vi "DimostratoreCalibrazioni.vi"() -> ()   [LabVIEW 2019]
uses:
  TypeDef/SlugExpiration.ctl
  ByteGSAPIBase/ByteGSAPIBase.lvclass
  TypeDef/CalibrationStates.ctl
  ByteGSAPIBase/FetchCalibration/Converted_Slug_Cluster.ctl
  ByteGSAPIBase/Instruments/Instruments.ctl
  ByteGSAPIBase/CalibrationMeasurements/BodyCalibrazioneMisure.ctl
  aa47c742-c095-4670-bf1f-6b28e4309cef.vi
  <vilib>/numeric/Random Number (Range) I64.vi
  <vilib>/Array/Sort 2D Array - Pop Stack.vi
  <vilib>/Array/Sort 2D Array - Push Stack.vi
  <vilib>/numeric/sub_Random U32.vi
panel:
  in  "Exit":bool
  out "Calibrations":string
  out "Status":string
  out "Calibration n.":string
  in  "Cancel":bool
  in  "Approvation":bool
  in  "Avanti":bool
  in  "Repeat":bool
  out "Outcome":string
  out "Measured value":dbl
  out "Reference value":dbl
  out "Waveform Chart":i64(graph)
  in  "Start Calibration":bool
  in  "Next":bool
  in  "Previus":bool
  out "Calibration n.":string
  in  "Filter":enum16{"All", "Expired", "Not Expired"}(ring)
  in  "Slug list":T1[](array[typedef])
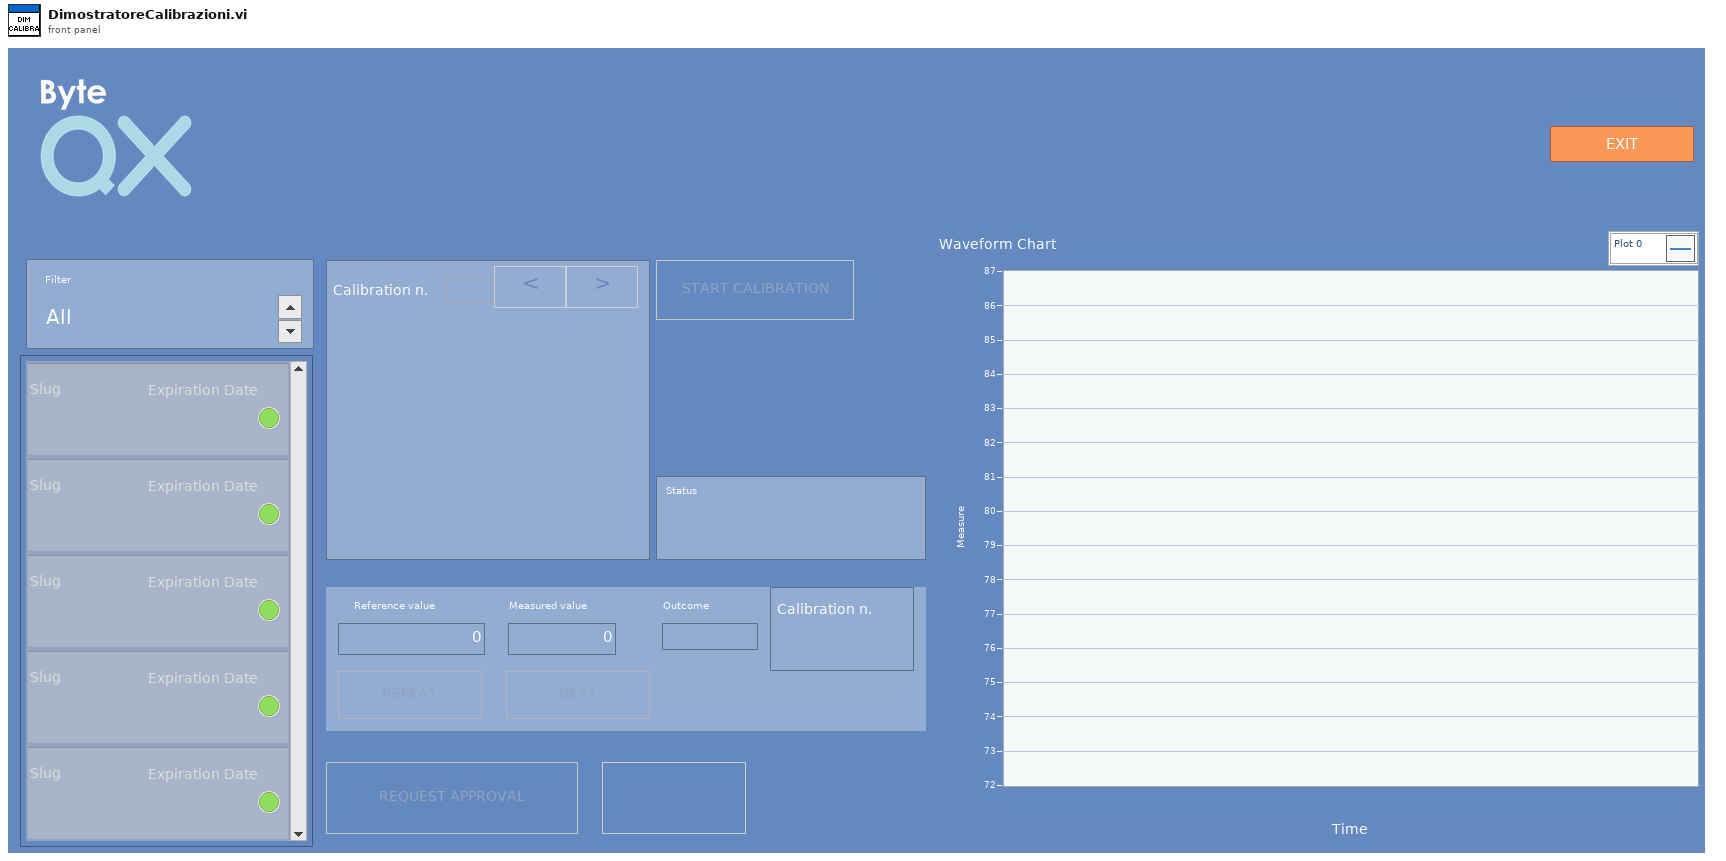
[diagram p1: front panel]
types:
  T1 = typedef "SlugExpiration.ctl" = cluster{"Slug":string, "Expiration Date":string, "Color Box":u32, "Active":bool, "Expired?":bool, "Id":i32}
  T2 = typedef "CalibrationStates.ctl" = enum16{"Init", "Idle", "GetInstruments", "Fetch", "GetCalibrations", "CheckTotalMisurations", "StartCalibration", "ManageCalibration", "AllowApprove", "Approve"}
  T3 = typedef "ByteGSWebAPI.lvlib/ByteGSAPIBase.lvclass/BodyCalibrazioneMisure.ctl" = cluster{"controls":cluster{"id":u16, "descrizione":string, "numero_misure_necessarie":u16, "riferimento_obiettivo":dbl, "mpe_max":dbl, "mpe_min":dbl, "deviazione_standard":dbl, "incertezza":dbl, "numero_misure_effettuate":u32, "temperatura_c":dbl, "umidita":dbl, "strumento_riferimento":cluster{"id":u16, "nome":string}[]}[]}
  T4 = typedef "Instruments.ctl" = cluster{"id":i32, "slug":string, "stabilimento":cluster{"id":dbl}, "categoria":cluster{"id":dbl}, "tipologia_di_visualizzazione":cluster{"id":dbl}, "stato":cluster{"id":dbl}, "descrizione":string, "costruttore":string, "matricola":string, "data_registrazione":string, "intervallo_di_taratura_mesi":dbl, "reparto":string, "campo_misura":string, "risoluzione":dbl, "responsabile_strumento":string, "classe_di_precisione":string, "classificazione":string, "appunti":string, "manuale":string, "foto":string, "riferimento":bool, "qr_hashcode":string, "costo_euro":dbl}
  T5 = typedef "ByteGSWebAPI.lvlib/ByteGSAPIBase.lvclass/Converted_Slug_Cluster.ctl" = cluster{"id":u32, "instrument":string, "name":string, "date":timestamp}
  T6 = cluster{"Outcome":refnum<vi>, "Avanti":refnum<vi>, "Repeat":refnum<vi>, "Slug list":refnum<vi>, "Start Calibration":refnum<vi>, "Avanti":refnum<vi>, "Cancel":refnum<vi>, "Approvation":refnum<vi>}
  T7 = cluster{"ByteGSAPIBase in":refnum<class "ByteGSAPIBase.lvclass">, "Instruments_Slug":string[], "All_Instruments_Cals":T5[], "All_Instruments":T4[], "Slug list All":T1[], "Calibrations":T3, "Selected Slug":i32, "Misurazioni":string, "Misurazioni index":i32, "Next State":T2, "Waveform Chart":refnum<vi>, "New Val":dbl, "Id Failed":u32, "Failed?":bool, "Cal Index":i32, "Misurazioni n":string, "Stato":string, "Esito":string, "Misure effettuate":i32, "Calibrations":string}
  T8 = cluster{"id":u16, "descrizione":string, "numero_misure_necessarie":u16, "riferimento_obiettivo":dbl, "mpe_max":dbl, "mpe_min":dbl, "deviazione_standard":dbl, "incertezza":dbl, "numero_misure_effettuate":u32, "temperatura_c":dbl, "umidita":dbl, "strumento_riferimento":cluster{"id":u16, "nome":string}[]}[]
  T9 = cluster{"id":u16, "descrizione":string, "numero_misure_necessarie":u16, "riferimento_obiettivo":dbl, "mpe_max":dbl, "mpe_min":dbl, "deviazione_standard":dbl, "incertezza":dbl, "numero_misure_effettuate":u32, "temperatura_c":dbl, "umidita":dbl, "strumento_riferimento":cluster{"id":u16, "nome":string}[]}
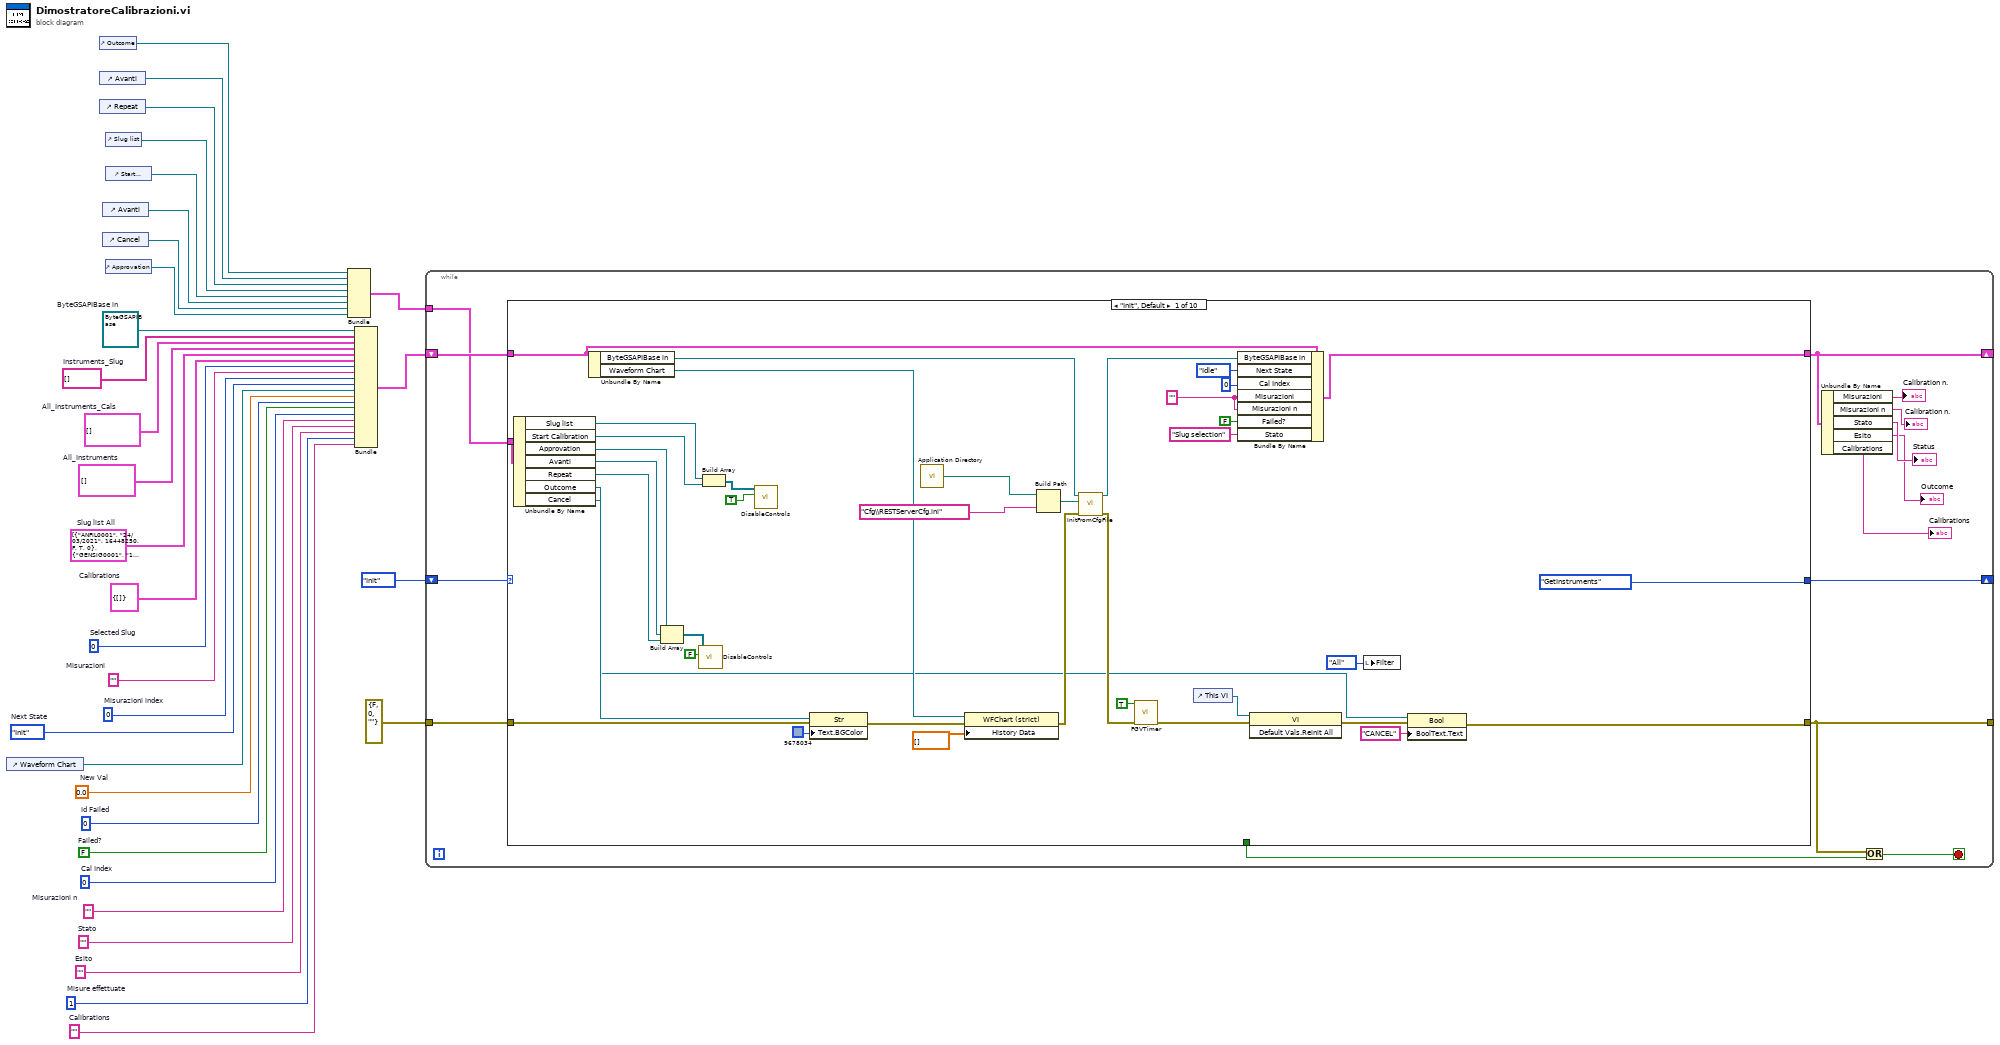
[diagram p0: block diagram]
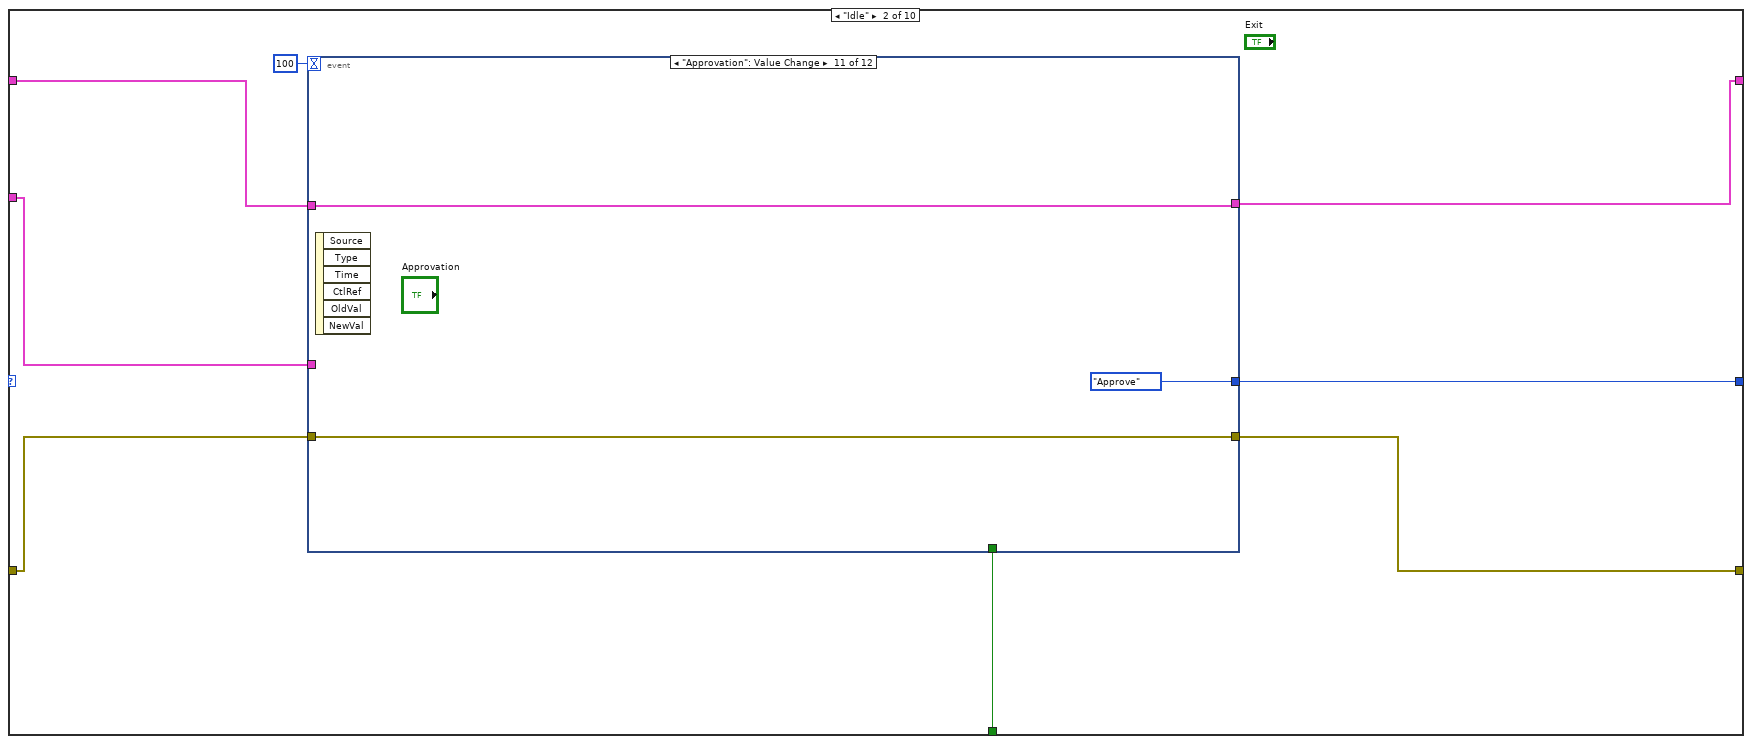
[diagram p2: hidden frame]
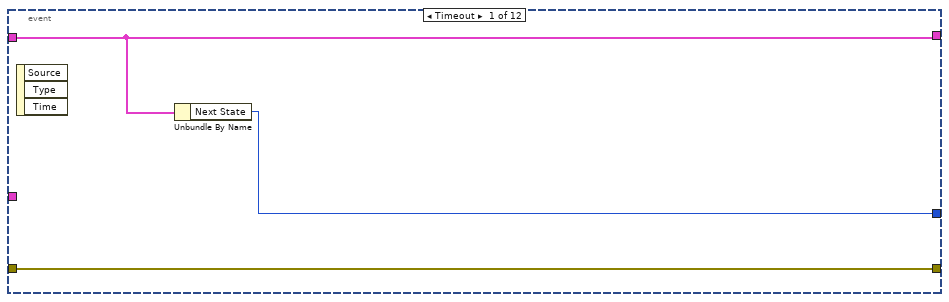
[diagram p3: hidden frame]
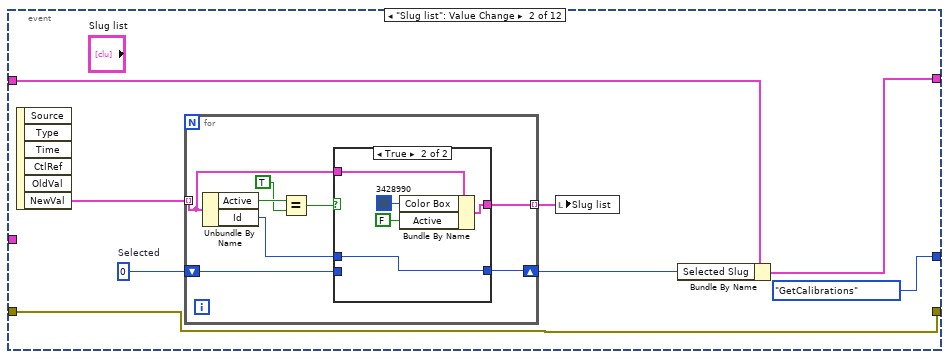
[diagram p4: hidden frame]
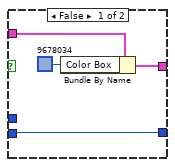
[diagram p5: hidden frame]
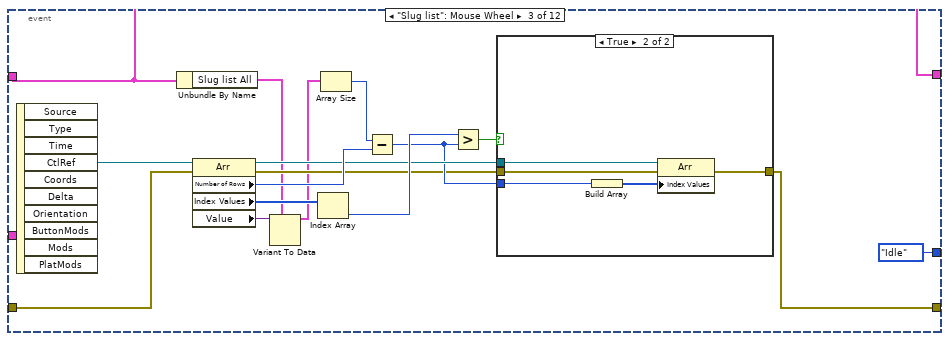
[diagram p6: hidden frame]
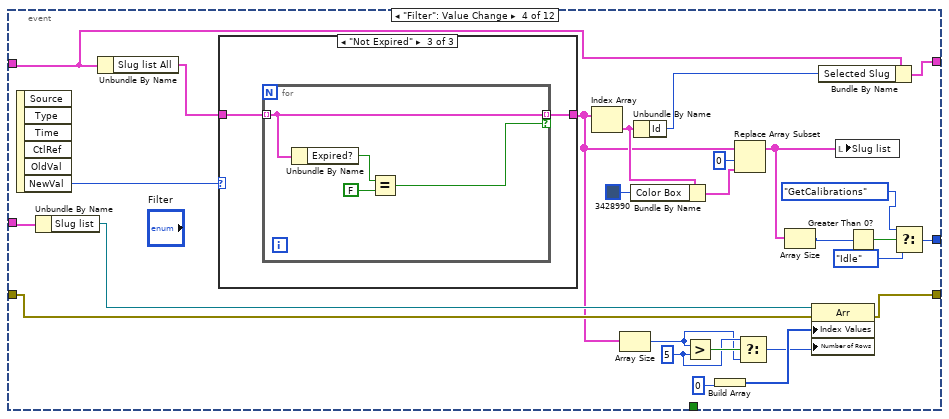
[diagram p8: hidden frame]
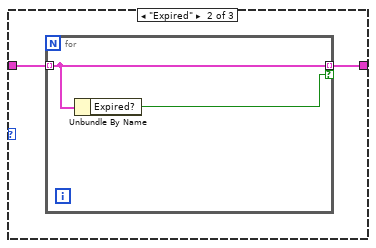
[diagram p10: hidden frame]
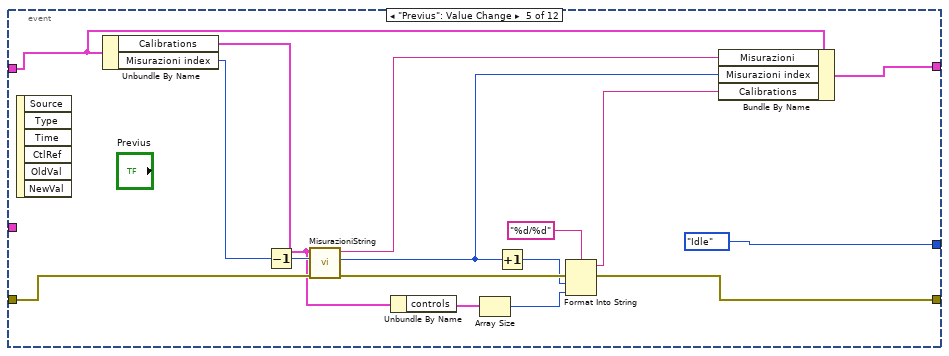
[diagram p11: hidden frame]
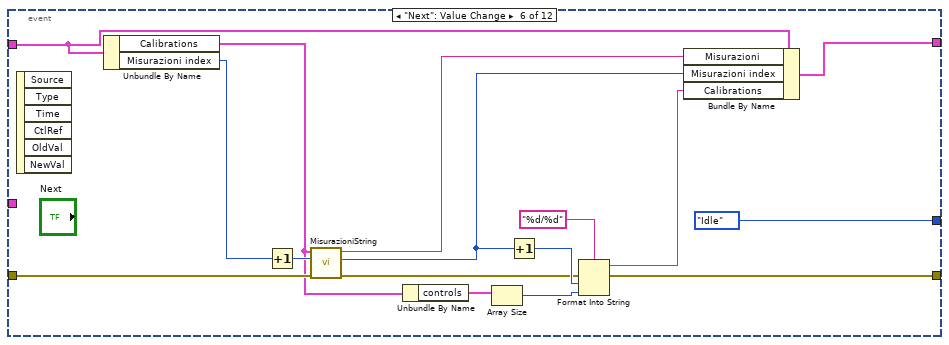
[diagram p12: hidden frame]
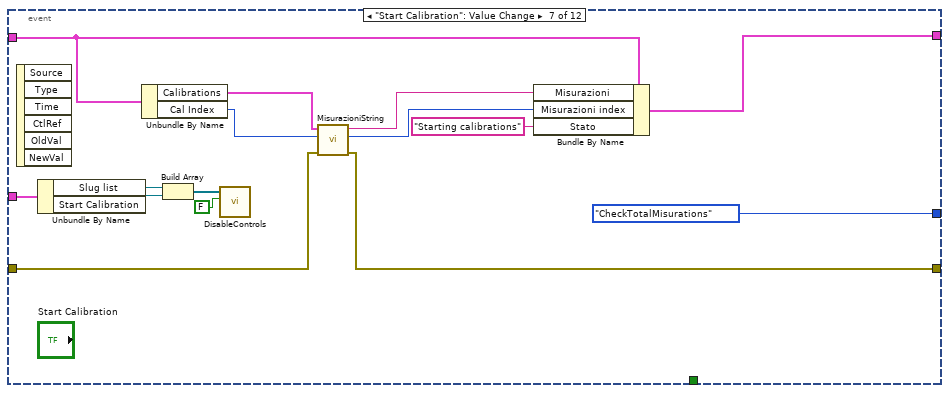
[diagram p13: hidden frame]
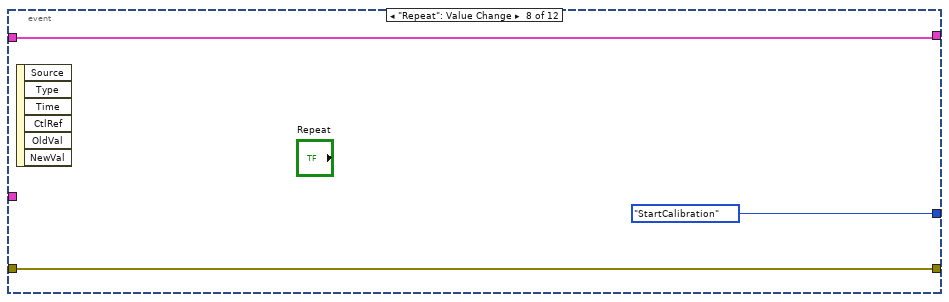
[diagram p14: hidden frame]
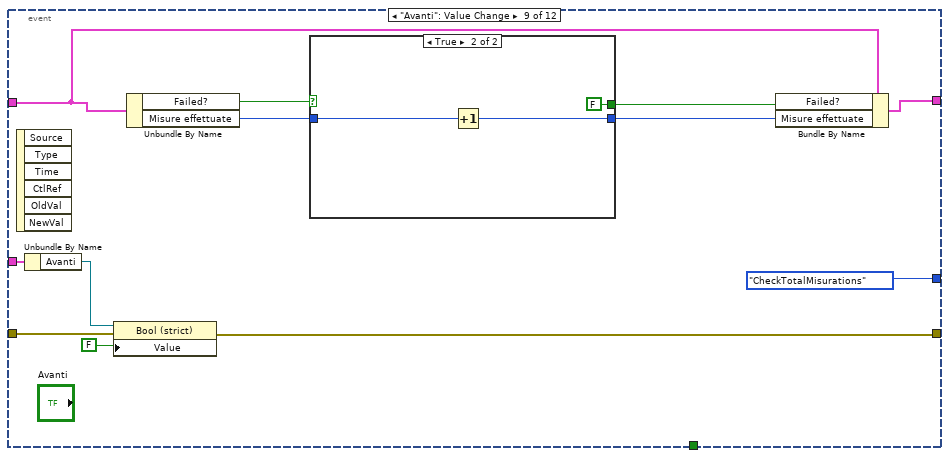
[diagram p15: hidden frame]
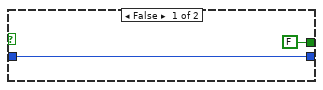
[diagram p16: hidden frame]
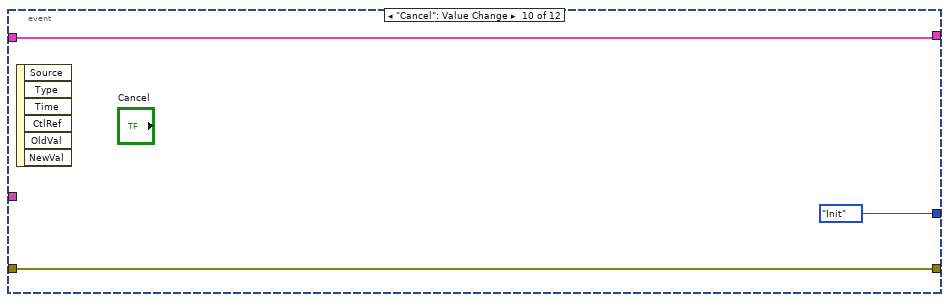
[diagram p17: hidden frame]
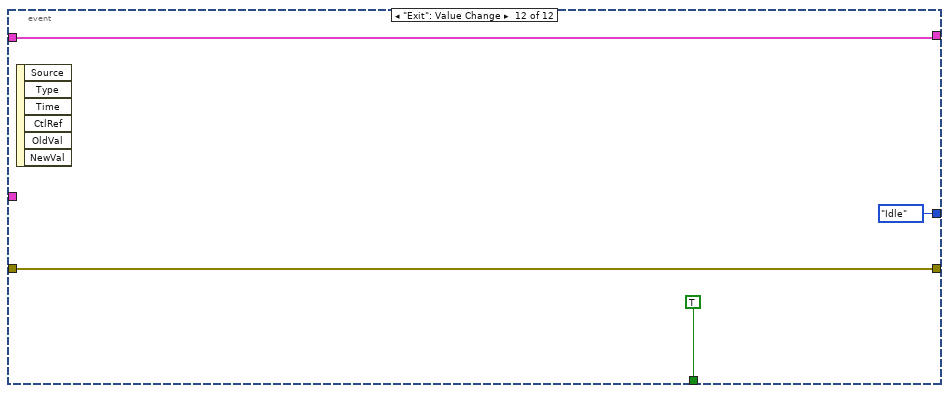
[diagram p18: hidden frame]
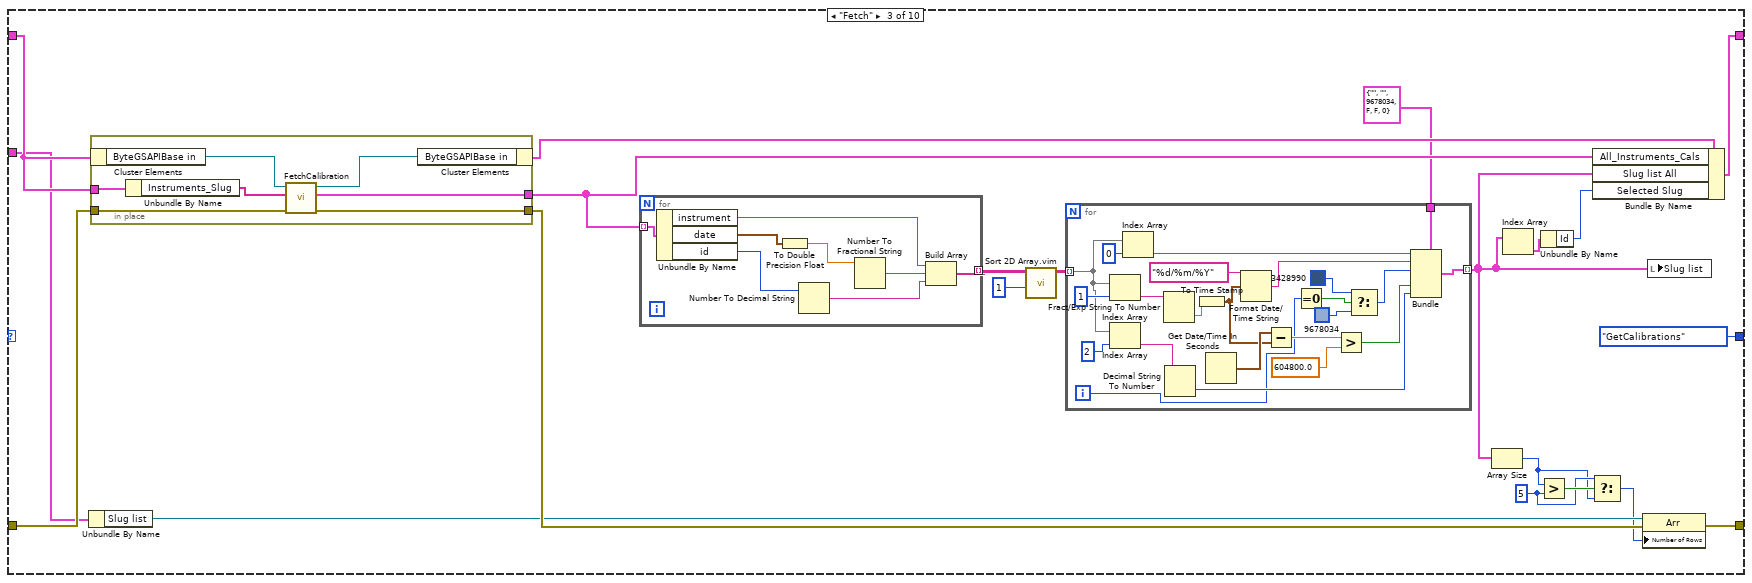
[diagram p19: hidden frame]
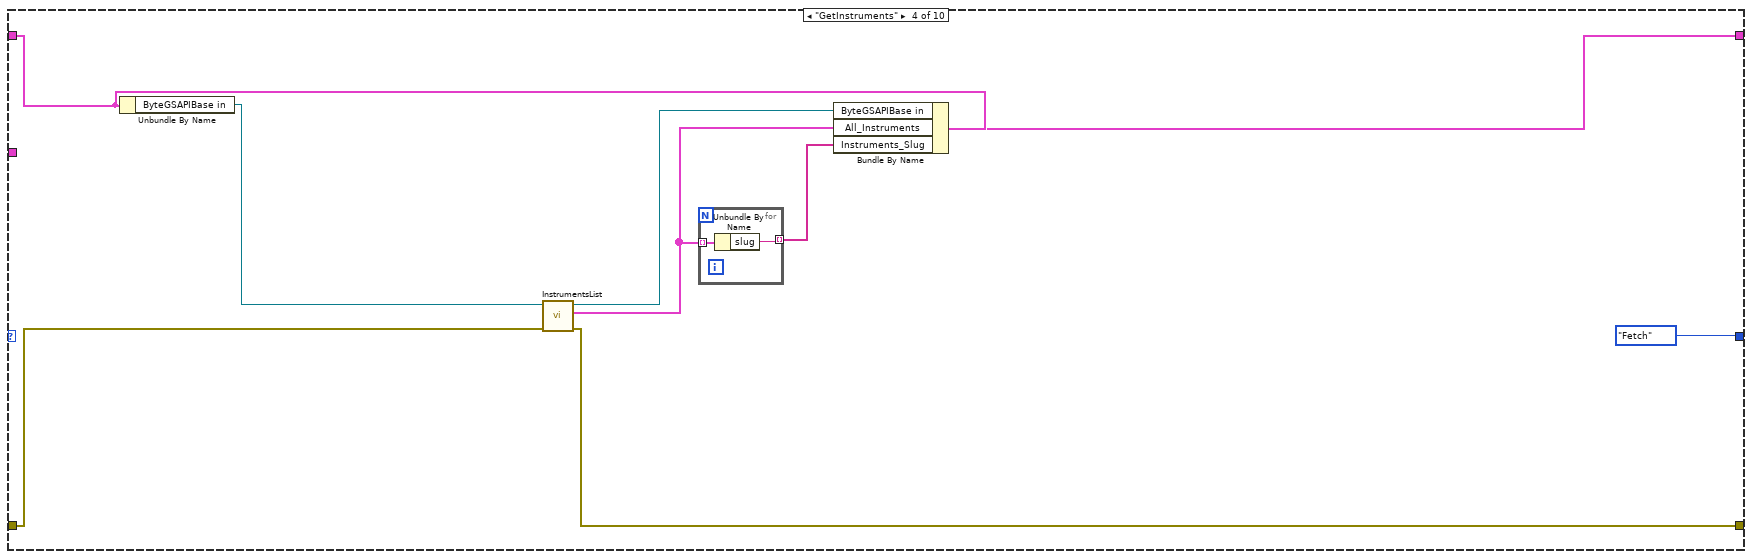
[diagram p20: hidden frame]
diagram:
  w1 = ""  # Calibrations
  w2 = 1  # Misure effettuate
  w4 = ""  # Esito
  w5 = ""  # Stato
  w10 = ""  # Misurazioni n
  w15 = 0  # Cal Index
  w16 = FALSE  # Failed?
  w17 = u32 0  # Id Failed
  w18 = 0.0  # New Val
  w20 = CalibrationStates."Init"  # Next State
  w21 = 0  # Misurazioni index
  w22 = ""  # Misurazioni
  w23 = T1[] [{"Slug"="ANFIL0001", "Expiration Date"="24/03/2021", "Color Box"=16448250, "Active"=FALSE, "Expired?"=TRUE, "Id"=0}, {"Slug"="GENSIG0001", "Expiration Date"="18/05/2021", "Color Box"=16448250, "Active"=FALSE, "Expired?"=TRUE, "Id"=0}, {"Slug"="GENSIG0001", "Expiration Date"="15/09/2021", "Color Box"=16448250, "Active"=FALSE, "Expired?"=TRUE, "Id"=0}, {"Slug"="DIN0001", "Expiration Date"="11/10/2021", "Color Box"=13816530, "Active"=FALSE, "Expired?"=TRUE, "Id"=0}, {"Slug"="DMM0002", "Expiration Date"="20/10/2021", "Color Box"=16448250, "Active"=FALSE, "Expired?"=TRUE, "Id"=0}, {"Slug"="COMP0001", "Expiration Date"="01/12/2021", "Color Box"=16448250, "Active"=FALSE, "Expired?"=TRUE, "Id"=0}, {"Slug"="TORS0002", "Expiration Date"="06/12/2021", "Color Box"=16448250, "Active"=FALSE, "Expired?"=TRUE, "Id"=0}, {"Slug"="CDIND0001", "Expiration Date"="04/03/2022", "Color Box"=16448250, "Active"=FALSE, "Expired?"=TRUE, "Id"=0}, {"Slug"="CALI0004", "Expiration Date"="11/03/2022", "Color Box"=16448250, "Active"=FALSE, "Expired?"=TRUE, "Id"=0}, {"Slug"="CALI0001", "Expiration Date"="10/05/2022", "Color Box"=16448250, "Active"=FALSE, "Expired?"=TRUE, "Id"=0}, {"Slug"="CALI0012", "Expiration Date"="10/05/2022", "Color Box"=16448250, "Active"=FALSE, "Expired?"=TRUE, "Id"=0}, {"Slug"="CALI0011", "Expiration Date"="11/05/2022", "Color Box"=16448250, "Active"=FALSE, "Expired?"=TRUE, "Id"=0}, {"Slug"="CALI0014", "Expiration Date"="04/07/2022", "Color Box"=16448250, "Active"=FALSE, "Expired?"=TRUE, "Id"=0}, {"Slug"="CDIND0001", "Expiration Date"="15/07/2022", "Color Box"=16448250, "Active"=FALSE, "Expired?"=TRUE, "Id"=0}, {"Slug"="CALI0024", "Expiration Date"="11/07/2023", "Color Box"=16448250, "Active"=FALSE, "Expired?"=TRUE, "Id"=0}, {"Slug"="CALI0017", "Expiration Date"="19/09/2023", "Color Box"=16448250, "Active"=FALSE, "Expired?"=TRUE, "Id"=0}, {"Slug"="CALI0020", "Expiration Date"="02/11/2023", "Color Box"=16448250, "Active"=FALSE, "Expired?"=TRUE, "Id"=0}, {"Slug"="CALI0017", "Expiration Date"="03/11/2023", "Color Box"=16448250, "Active"=FALSE, "Expired?"=TRUE, "Id"=0}, {"Slug"="CALI0025", "Expiration Date"="11/11/2023", "Color Box"=16448250, "Active"=FALSE, "Expired?"=TRUE, "Id"=0}, {"Slug"="CLBR0001", "Expiration Date"="30/11/2023", "Color Box"=16448250, "Active"=FALSE, "Expired?"=TRUE, "Id"=0}, {"Slug"="CLBR0001", "Expiration Date"="02/01/2024", "Color Box"=16448250, "Active"=FALSE, "Expired?"=TRUE, "Id"=0}, {"Slug"="CLBR0001", "Expiration Date"="02/01/2024", "Color Box"=16448250, "Active"=FALSE, "Expired?"=TRUE, "Id"=0}, {"Slug"="CLBR0003", "Expiration Date"="04/03/2024", "Color Box"=16448250, "Active"=FALSE, "Expired?"=TRUE, "Id"=0}, {"Slug"="MICP0001", "Expiration Date"="19/03/2024", "Color Box"=16448250, "Active"=FALSE, "Expired?"=TRUE, "Id"=0}, {"Slug"="TERM0002", "Expiration Date"="04/07/2024", "Color Box"=16448250, "Active"=FALSE, "Expired?"=TRUE, "Id"=0}, {"Slug"="ACCEL0008", "Expiration Date"="04/07/2024", "Color Box"=16448250, "Active"=FALSE, "Expired?"=TRUE, "Id"=0}, {"Slug"="ACCEL0008", "Expiration Date"="05/07/2024", "Color Box"=16448250, "Active"=FALSE, "Expired?"=TRUE, "Id"=0}, {"Slug"="ACCEL0008", "Expiration Date"="19/08/2024", "Color Box"=16448250, "Active"=FALSE, "Expired?"=TRUE, "Id"=0}, {"Slug"="TERM0002", "Expiration Date"="15/10/2024", "Color Box"=16448250, "Active"=FALSE, "Expired?"=TRUE, "Id"=0}, {"Slug"="BILA0001", "Expiration Date"="15/10/2024", "Color Box"=16448250, "Active"=FALSE, "Expired?"=TRUE, "Id"=0}, {"Slug"="CLBR0001", "Expiration Date"="15/10/2024", "Color Box"=16448250, "Active"=FALSE, "Expired?"=TRUE, "Id"=0}, {"Slug"="ACCEL0002", "Expiration Date"="15/10/2024", "Color Box"=16448250, "Active"=FALSE, "Expired?"=TRUE, "Id"=0}]  # Slug list All
  w24 = 0  # Selected Slug
  w25 = T3 {"controls"=[]}  # Calibrations
  w26 = T4[] []  # All_Instruments
  w27 = T5[] []  # All_Instruments_Cals
  w28 = string[] []  # Instruments_Slug
  w31 = refnum<class "ByteGSAPIBase.lvclass"> refnum  # ByteGSAPIBase in
  n1 = control-ref of="Waveform Chart"() -> (w19:refnum<vi>)
  n2 = control-ref of="Avanti"() -> (w6:refnum<vi>)
  n3 = control-ref of="Repeat"() -> (w7:refnum<vi>)
  n4 = control-ref of="Outcome"() -> (w3:refnum<vi>)
  n5 = control-ref of="Avanti"() -> (w11:refnum<vi>)
  n6 = control-ref of="Cancel"() -> (w12:refnum<vi>)
  n7 = control-ref of="Start Calibration"() -> (w9:refnum<vi>)
  n8 = control-ref of="Approvation"() -> (w13:refnum<vi>)
  n9 = control-ref of="Slug list"() -> (w8:refnum<vi>)
  n10 = Bundle("Outcome"=w3, "Avanti"=w6, "Repeat"=w7, "Slug list"=w8, "Start Calibration"=w9, "Avanti"=w11, "Cancel"=w12, "Approvation"=w13) -> (w14:T6)  [unwired: 1 in]
  n11 = Bundle("ByteGSAPIBase in"=w31, "Instruments_Slug"=w28, "All_Instruments_Cals"=w27, "All_Instruments"=w26, "Slug list All"=w23, "Calibrations"=w25, "Selected Slug"=w24, "Misurazioni"=w22, "Misurazioni index"=w21, "Next State"=w20, "Waveform Chart"=w19, "New Val"=w18, "Id Failed"=w17, "Failed?"=w16, "Cal Index"=w15, "Misurazioni n"=w10, "Stato"=w5, "Esito"=w4, "Misure effettuate"=w2, "Calibrations"=w1) -> (w30:T7)  [unwired: 1 in]
  n12 = while {
    shift-right: [w45] -> _
    shift-left: CalibrationStates."Init" -> [w46]
    shift-right: [w42] -> _
    shift-left: w30 -> [w44]
    tunnel: w14 -> [w40]
    tunnel: errorcluster {"status"=FALSE, "code"=0, "source"=""} ("error in (no error)") -> [w43]
    tunnel: [w33] -> _
    stop <- w35 stop-if-true
    n13 = case shown="\"Init\", Default" w46 {
      tunnel: [CalibrationStates."GetInstruments" w91 CalibrationStates."GetCalibrations" CalibrationStates."Fetch" CalibrationStates."Idle" w371 CalibrationStates."Idle" CalibrationStates."Idle" CalibrationStates."Idle" CalibrationStates."Idle"] -> w45
      tunnel: w44 -> [w81 w93 w278 w323 w352 w367 w443 w479 w546 w583]
      tunnel: w43 -> [w53 w90 w277 w325 w353 w369 w428 w465 w549 w582]
      tunnel: [w48 w89 w264 w319 w345 w368 w418 w466 w549 w571] -> w33
      tunnel: [w79 w92 w274 w321 w351 w366 w442 w478 w546 w575] -> w42
      tunnel: w40 -> [w69 w87 w265 _ w338 w370 w432 w471 w555 w580]
      tunnel: [_ w86 _ _ _ _ _ _ _ _] -> w34
      frame "Init", Default {
        w66 = "" ("Misurazioni")
        n14 = Unbundle By Name(w69) -> ("Slug list"=w65:refnum<vi>, "Start Calibration"=w64:refnum<vi>, "Approvation"=w47:refnum<vi>, "Avanti"=w59:refnum<vi>, "Repeat"=w58:refnum<vi>, "Outcome"=w52:refnum<vi>, "Cancel"=w50:refnum<vi>)
        n15 = Unbundle By Name(w81) -> ("ByteGSAPIBase in"=w82:refnum<class "ByteGSAPIBase.lvclass">, "Waveform Chart"=w73:refnum<vi>)
        n16 = Build Array(w47, w59, w58) -> (w61:refnum<vi>[])
        n17 = call "DisableControls.vi"("Visible"=FALSE, "Controls"=w61) -> ()  [unwired: 9 in, 1 out]
        n18 = Build Array(w65, w64) -> (w63:refnum<vi>[])
        n19 = call "DisableControls.vi"("Visible"=TRUE, "Controls"=w63) -> ()  [unwired: 9 in, 1 out]
        n20 = property class="Str"(reference=w52, error in=w53, "Text.BGColor"=u32 9678034 ("Text.Text Colors:BG Color")) -> (error out=w54:errorcluster)  [unwired: 1 out]
        n21 = call <vilib>:"Application Directory.vi"() -> ("Application Directory"=w83:path)
        n22 = property class="WFChart (strict)"(reference=w73, error in=w54, "History Data"=dbl[] []) -> (error out=w72:errorcluster)  [unwired: 1 out]
        n23 = Build Path(base path=w83, name or relative path="Cfg\\RESTServerCfg.ini") -> (appended path=w78:path)
        n24 = call-dynamic "InitFromCfgFile.vi"("error in (no error)"=w72, "configuration file path"=w78, "ByteGSAPIBase in"=w82) -> ("error out"=w76:errorcluster, "ByteGSAPIBase out"=w80:refnum<class "ByteGSAPIBase.lvclass">)  [unwired: 7 in]
        n25 = call "FGVTimer.vi"("error in"=w76, "Reset"=TRUE) -> ("error out"=w68:errorcluster)  [unwired: 7 in, 2 out]
        n26 = control-ref of="This VI"() -> (w67:refnum<vi>)
        n27 = Bundle By Name(cluster=w81, "ByteGSAPIBase in"=w80, "Next State"=CalibrationStates."Idle", "Cal Index"=0, "Misurazioni"=w66, "Misurazioni n"=w66, "Failed?"=FALSE, "Stato"="Slug selection") -> (w79:T7)
        n28 = invoke class="VI" method="Default Vals.Reinit All"(reference=w67, error in=w68) -> (error out=w51:errorcluster)  [unwired: 1 in, 2 out]
        n29 = local write "Filter"(enum16{"All", "Expired", "Not Expired"}."All" ("Filter")) -> ()
        n30 = property class="Bool"(reference=w50, error in=w51, "BoolText.Text"="CANCEL" ("Boolean Text.Text")) -> (error out=w48:errorcluster)  [unwired: 1 out]
      }
      frame "Idle" {
        n31 = event shown="[10] \"Approvation\": Value Change" {
          selector: _ -> [_ _ _ _ _ _ _ _ _ _ _ _]
          dyn-events: _ -> [_ _ _ _ _ _ _ _ _ _ _ _]
          timeout: 100 -> [_ _ _ _ _ _ _ _ _ _ _ _]
          tunnel: w93 -> [w95 w101 w125 w167 w193 w209 w224 w230 w234 w248 w251 w254]
          tunnel: [w95 w99 w125 w166 w192 w207 w221 w230 w233 w248 w251 w254] -> w92
          tunnel: [w94 CalibrationStates."GetCalibrations" CalibrationStates."Idle" w144 CalibrationStates."Idle" CalibrationStates."Idle" CalibrationStates."CheckTotalMisurations" CalibrationStates."StartCalibration" CalibrationStates."CheckTotalMisurations" CalibrationStates."Init" CalibrationStates."Approve" CalibrationStates."Idle"] -> w91
          tunnel: w90 -> [w96 w97 w129 w157 w190 w212 w220 w228 w237 w250 w253 w256]
          tunnel: [w96 w97 w127 w156 w188 w198 w218 w228 w238 w250 w253 w256] -> w89
          tunnel: w87 -> [_ _ _ w159 _ _ w219 _ w239 _ _ _]
          tunnel: [_ _ _ _ _ _ _ _ _ _ _ TRUE] -> w86
          event Timeout {
            n32 = event-data() -> ()  [unwired: 1 in, 3 out]
            n33 = Unbundle By Name(w95) -> ("Next State"=w94:T2)
          }
          event "Slug list": Value Change {
            w102 = 0  # Selected
            n34 = event-data() -> ("NewVal"=w104:T1[])  [unwired: 1 in, 5 out]
            n35 = for {
              tunnel: w104 -> [w109] mode=indexing
              tunnel: [w108] -> w103 mode=indexing
              shift-right: [w106] -> w100
              shift-left: w102 -> [w107]
              n36 = Unbundle By Name(w109) -> ("Active"=w112:bool, "Id"=w105:i32)
              n37 = Equal?(x=w112, y=TRUE) -> (x = y?=w110:bool)
              n38 = case shown="True" w110 {
                tunnel: w109 -> [w115 w121]
                tunnel: [w116 w119] -> w108
                tunnel: w107 -> [w113 _]
                tunnel: [w113 w117] -> w106
                tunnel: w105 -> [_ w117]
                frame False {
                  n39 = Bundle By Name(cluster=w115, "Color Box"=u32 9678034) -> (w116:T1)
                }
                frame True {
                  n40 = Bundle By Name(cluster=w121, "Color Box"=u32 3428990, "Active"=FALSE) -> (w119:T1)
                }
              }
            }
            n41 = local write "Slug list"(w103) -> ()
            n42 = Bundle By Name(cluster=w101, "Selected Slug"=w100) -> (w99:T7)
          }
          event "Slug list": Mouse Wheel {
            n43 = event-data() -> ("CtlRef"=w137:refnum<vi>)  [unwired: 1 in, 9 out]
            n44 = Unbundle By Name(w125) -> ("Slug list All"=w122:T1[])
            n45 = property class="Arr"(reference=w137, error in=w129) -> (reference out=w131:refnum<vi>, error out=w128:errorcluster, "Number of Rows"=w134:u32, "Index Values"=w136:u32[], "Value"=w123:variant)
            n46 = Variant To Data(type=w122, Variant=w123) -> (data=w124:T1[])  [unwired: 1 in, 1 out]
            n47 = Index Array(array=w136) -> (element=w133:u32)  [unwired: 1 in]
            n48 = Array Size(array=w124) -> (size(s)=w135:i32)
            n49 = Subtract(x=w135, y=w134) -> (x-y=w130:u32)
            n50 = Greater?(x=w133, y=w130) -> (0:w132:bool)
            n51 = case shown="True" w132 {
              tunnel: w131 -> [_ w143]
              tunnel: w130 -> [_ w142]
              tunnel: w128 -> [w138 w140]
              tunnel: [w138 w139] -> w127
              frame False {
              }
              frame True {
                n52 = Build Array(w142) -> (w141:u32[])
                n53 = property class="Arr"(reference=w143, error in=w140, "Index Values"=w141) -> (error out=w139:errorcluster)  [unwired: 1 out]
              }
            }
          }
          event "Filter": Value Change {
            w153 = 5 ("y")
            n54 = event-data() -> ("NewVal"=w169:enum16{"All", "Expired", "Not Expired"})  [unwired: 1 in, 5 out]
            n55 = Unbundle By Name(w159) -> ("Slug list"=w158:refnum<vi>)
            n56 = Unbundle By Name(w167) -> ("Slug list All"=w168:T1[])
            n57 = case shown="\"Not Expired\"" w169 {
              tunnel: w168 -> [w170 w172 w176]
              tunnel: [w170 w171 w175] -> w150
              frame "All" {
              }
              frame "Expired" {
                n58 = for {
                  tunnel: w172 -> [w174] mode=indexing
                  tunnel: [w174] -> w171 mode=indexing if=w173
                  n59 = Unbundle By Name(w174) -> ("Expired?"=w173:bool)
                }
              }
              frame "Not Expired" {
                n60 = for {
                  tunnel: w176 -> [w180] mode=indexing
                  tunnel: [w180] -> w175 mode=indexing if=w177
                  n61 = Unbundle By Name(w180) -> ("Expired?"=w179:bool)
                  n62 = Equal?(x=w179, y=FALSE) -> (x = y?=w177:bool)
                }
              }
            }
            n63 = Index Array(array=w150) -> (element=w164:T1)  [unwired: 1 in]
            n64 = Array Size(array=w150) -> (size(s)=w152:i32)
            n65 = Bundle By Name(cluster=w164, "Color Box"=u32 3428990) -> (w162:T1)
            n66 = Unbundle By Name(w164) -> ("Id"=w165:i32)
            n67 = Greater?(x=w152, y=w153) -> (0:w154:bool)
            n68 = Build Array(0) -> (w160:i32[])
            n69 = Replace Array Subset(array=w150, new element=w162, index=0) -> (w147:T1[])
            n70 = Select(t=w153, s=w154, f=w152) -> (s? t:f=w151:i32)
            n71 = Array Size(array=w147) -> (size(s)=w148:i32)
            n72 = property class="Arr"(reference=w158, error in=w157, "Index Values"=w160, "Number of Rows"=w151) -> (error out=w156:errorcluster)  [unwired: 1 out]
            n73 = Bundle By Name(cluster=w167, "Selected Slug"=w165) -> (w166:T7)
            n74 = local write "Slug list"(w147) -> ()
            n75 = Greater Than 0?(x=w148) -> (x > 0?=w149:bool)
            n76 = Select(t=CalibrationStates."GetCalibrations", s=w149, f=CalibrationStates."Idle") -> (s? t:f=w144:T2)
          }
          event "Previus": Value Change {
            n77 = event-data() -> ()  [unwired: 1 in, 6 out]
            n78 = Unbundle By Name(w193) -> ("Calibrations"=w184:T3, "Misurazioni index"=w195:i32)
            n79 = Decrement(x=w195) -> (x-1=w196:i32)
            n80 = call "MisurazioniString.vi"("error in (no error)"=w190, "index"=w196, "Calibration data"=w184) -> ("error out"=w189:errorcluster, "index"=w186:i32, "String"=w194:string)  [unwired: 6 in]
            n81 = Unbundle By Name(w184) -> ("controls"=w183:T8)
            n82 = Array Size(array=w183) -> (size(s)=w182:i32)
            n83 = Increment(x=w186) -> (x+1=w185:i32)
            n84 = Format Into String(format string="%d/%d", error in=w189, w185, w182) -> (resulting string=w181:string, error out=w188:errorcluster)  [unwired: 1 in]
            n85 = Bundle By Name(cluster=w193, "Misurazioni"=w194, "Misurazioni index"=w186, "Calibrations"=w181) -> (w192:T7)
          }
          event "Next": Value Change {
            n86 = event-data() -> ()  [unwired: 1 in, 6 out]
            n87 = Unbundle By Name(w209) -> ("Calibrations"=w203:T3, "Misurazioni index"=w210:i32)
            n88 = Increment(x=w210) -> (x+1=w211:i32)
            n89 = call "MisurazioniString.vi"("error in (no error)"=w212, "index"=w211, "Calibration data"=w203) -> ("error out"=w201:errorcluster, "index"=w200:i32, "String"=w208:string)  [unwired: 6 in]
            n90 = Unbundle By Name(w203) -> ("controls"=w199:T8)
            n91 = Array Size(array=w199) -> (size(s)=w202:i32)
            n92 = Increment(x=w200) -> (x+1=w204:i32)
            n93 = Format Into String(format string="%d/%d", error in=w201, w204, w202) -> (resulting string=w197:string, error out=w198:errorcluster)  [unwired: 1 in]
            n94 = Bundle By Name(cluster=w209, "Misurazioni"=w208, "Misurazioni index"=w200, "Calibrations"=w197) -> (w207:T7)
          }
          event "Start Calibration": Value Change {
            n95 = event-data() -> ()  [unwired: 1 in, 6 out]
            n96 = Unbundle By Name(w219) -> ("Slug list"=w217:refnum<vi>, "Start Calibration"=w216:refnum<vi>)
            n97 = Unbundle By Name(w224) -> ("Calibrations"=w226:T3, "Cal Index"=w225:i32)
            n98 = Build Array(w217, w216) -> (w215:refnum<vi>[])
            n99 = call "DisableControls.vi"("Visible"=FALSE, "Controls"=w215) -> ()  [unwired: 9 in, 1 out]
            n100 = call "MisurazioniString.vi"("error in (no error)"=w220, "index"=w225, "Calibration data"=w226) -> ("error out"=w218:errorcluster, "index"=w222:i32, "String"=w223:string)  [unwired: 6 in]
            n101 = Bundle By Name(cluster=w224, "Misurazioni"=w223, "Misurazioni index"=w222, "Stato"="Starting calibrations") -> (w221:T7)
          }
          event "Repeat": Value Change {
            n102 = event-data() -> ()  [unwired: 1 in, 6 out]
          }
          event "Avanti": Value Change {
            n103 = event-data() -> ()  [unwired: 1 in, 6 out]
            n104 = Unbundle By Name(w239) -> ("Avanti"=w241:refnum<vi>)
            n105 = property class="Bool (strict)"(reference=w241, error in=w237, "Value"=FALSE) -> (error out=w238:errorcluster)  [unwired: 1 out]
            n106 = Unbundle By Name(w234) -> ("Failed?"=w236:bool, "Misure effettuate"=w235:i32)
            n107 = case shown="True" w236 {
              tunnel: w235 -> [w244 w247]
              tunnel: [w244 w246] -> w232
              tunnel: [FALSE FALSE] -> w231
              frame False {
              }
              frame True {
                n108 = Increment(x=w247) -> (x+1=w246:i32)
              }
            }
            n109 = Bundle By Name(cluster=w234, "Failed?"=w231, "Misure effettuate"=w232) -> (w233:T7)
          }
          event "Cancel": Value Change {
            n110 = event-data() -> ()  [unwired: 1 in, 6 out]
          }
          event "Approvation": Value Change {
            n111 = event-data() -> ()  [unwired: 1 in, 6 out]
          }
          event "Exit": Value Change {
            n112 = event-data() -> ()  [unwired: 1 in, 6 out]
          }
        }
      }
      frame "Fetch" {
        w260 = 5 ("y")
        n113 = Unbundle By Name(w265) -> ("Slug list"=w262:refnum<vi>)
        n114 = in-place {
          in-place-border: w277 -> [w315]
          in-place-border: [w314] -> w263
          in-place-border: [w313] -> w270
          in-place-border: w278 -> [w311]
          n115 = in-place-cluster #1(w278) -> ("ByteGSAPIBase in"=w312:refnum<class "ByteGSAPIBase.lvclass">)
          n116 = Unbundle By Name(w311) -> ("Instruments_Slug"=w310:string[])
          n117 = call-dynamic "FetchCalibration.vi"("error in (no error)"=w315, "instruments"=w310, "ByteGSAPIBase in"=w312) -> ("error out"=w314:errorcluster, "instruments"=w313:T5[], "ByteGSAPIBase out"=w316:refnum<class "ByteGSAPIBase.lvclass">)  [unwired: 6 in]
          n118 = in-place-cluster #1("ByteGSAPIBase in"=w316) -> (w275:T7)
        }
        n119 = for {
          tunnel: w270 -> [w309] mode=indexing
          tunnel: [w308] -> w273 mode=indexing
          n120 = Unbundle By Name(w309) -> ("instrument"=w307:string, "date"=w306:timestamp, "id"=w303:u32)
          n121 = To Double Precision Float(number=w306) -> (double precision float=w305:dbl)
          n122 = Number To Decimal String(number=w303) -> (decimal integer string=w302:string)  [unwired: 1 in]
          n123 = Number To Fractional String(number=w305) -> (F-format string=w304:string)  [unwired: 3 in]
          n124 = Build Array(w307, w304, w302) -> (w308:string[])
        }
        n125 = call "Sort 2D Array.vim"("index"=1, "2D array"=w273) -> ("sorted 2D array"=w271:string[][])  [unwired: 8 in, 1 out]
        n126 = for {
          tunnel: w271 -> [w286] mode=indexing
          tunnel: T1 {"Slug"="", "Expiration Date"="", "Color Box"=9678034, "Active"=FALSE, "Expired?"=FALSE, "Id"=0} ("Slug list 2") -> [w301]
          tunnel: [w293] -> w266 mode=indexing
          i -> [w283]
          n127 = Index Array(array=w286, index=1) -> (element=w297:string)
          n128 = Index Array(array=w286, index=2) -> (element=w285:string)
          n129 = Index Array(array=w286, index=0) -> (element=w299:string)
          n130 = Fract/Exp String To Number(string=w297) -> (number=w296:dbl)  [unwired: 3 in, 1 out]
          n131 = Decimal String To Number(string=w285) -> (number=w284:i32)  [unwired: 2 in, 1 out]
          n132 = To Time Stamp(1:w296) -> (0:w288:timestamp)
          n133 = Get Date/Time In Seconds() -> (seconds since 1Jan1904=w289:timestamp)
          n134 = Format Date/Time String(time format string (%c)="%d/%m/%Y", seconds (now)=w288) -> (date/time string=w294:string)  [unwired: 1 in]
          n135 = Subtract(x=w289, y=w288) -> (x-y=w292:dbl)
          n136 = Equal To 0?(x=w283) -> (x = 0?=w282:bool)
          n137 = Greater?(x=w292, y=604800.0) -> (0:w290:bool)
          n138 = Select(t=u32 3428990 ("Color Box"), s=w282, f=u32 9678034 ("Color Box")) -> (s? t:f=w279:u32)
          n139 = Bundle(cluster=w301, "Slug"=w299, "Expiration Date"=w294, "Color Box"=w279, "Expired?"=w290, "Id"=w284) -> (w293:T1)  [unwired: 1 in]
        }
        n140 = Array Size(array=w266) -> (size(s)=w259:i32)
        n141 = Index Array(array=w266) -> (element=w268:T1)  [unwired: 1 in]
        n142 = Greater?(x=w259, y=w260) -> (0:w261:bool)
        n143 = Unbundle By Name(w268) -> ("Id"=w267:i32)
        n144 = Select(t=w260, s=w261, f=w259) -> (s? t:f=w258:i32)
        n145 = Bundle By Name(cluster=w275, "All_Instruments_Cals"=w270, "Slug list All"=w266, "Selected Slug"=w267) -> (w274:T7)
        n146 = property class="Arr"(reference=w262, error in=w263, "Number of Rows"=w258) -> (error out=w264:errorcluster)  [unwired: 1 out]
        n147 = local write "Slug list"(w266) -> ()
      }
      frame "GetInstruments" {
        n148 = Unbundle By Name(w323) -> ("ByteGSAPIBase in"=w324:refnum<class "ByteGSAPIBase.lvclass">)
        n149 = call "InstrumentsList.vi"("error in (no error)"=w325, "ByteGSAPIBase in"=w324) -> ("error out"=w319:errorcluster, "Array"=w318:T4[], "ByteGSAPIBase out"=w322:refnum<class "ByteGSAPIBase.lvclass">)  [unwired: 7 in]
        n150 = for {
          tunnel: w318 -> [w327] mode=indexing
          tunnel: [w326] -> w317 mode=indexing
          n151 = Unbundle By Name(w327) -> ("slug"=w326:string)
        }
        n152 = Bundle By Name(cluster=w323, "ByteGSAPIBase in"=w322, "All_Instruments"=w318, "Instruments_Slug"=w317) -> (w321:T7)
      }
      frame "GetCalibrations" {
        n153 = Unbundle By Name(w338) -> ("Start Calibration"=w335:refnum<vi>)
        n154 = Unbundle By Name(w352) -> ("ByteGSAPIBase in"=w354:refnum<class "ByteGSAPIBase.lvclass">, "Selected Slug"=w355:i32)
        n155 = call-dynamic "ExecutingCalibration.vi"("error in (no error)"=w353, "calibration_id"=w355, "ByteGSAPIBase in"=w354) -> ("error out"=w349:errorcluster, "calibration data"=w346:T3, "ByteGSAPIBase out"=w350:refnum<class "ByteGSAPIBase.lvclass">)  [unwired: 6 in]
        n156 = call "MisurazioniString.vi"("error in (no error)"=w349, "index"=0, "Calibration data"=w346) -> ("error out"=w329:errorcluster, "index"=w332:i32, "String"=w348:string)  [unwired: 6 in]
        n157 = Unbundle By Name(w346) -> ("controls"=w339:T8)
        n158 = for {
          tunnel: w339 -> [w363] mode=indexing
          tunnel: [w357] -> w336
          stop <- w357 stop-if-true
          n159 = Unbundle By Name(w363) -> ("numero_misure_necessarie"=w362:u16, "numero_misure_effettuate"=w361:u32)
          n160 = Less Or Equal?(x=w362, y=w361) -> (x <= y?=w360:bool)
          n161 = Select(t=FALSE, s=w360, f=TRUE) -> (s? t:f=w357:bool)
        }
        n162 = Build Array(w335) -> (w337:refnum<vi>[])
        n163 = call "DisableControls.vi"("Visible"=w336, "Controls"=w337) -> ()  [unwired: 9 in, 1 out]
        n164 = Index Array(array=w339) -> (element=w342:T9)  [unwired: 1 in]
        n165 = Array Size(array=w339) -> (size(s)=w333:i32)
        n166 = Increment(x=w332) -> (x+1=w331:i32)
        n167 = Unbundle By Name(w342) -> ("numero_misure_effettuate"=w340:u32, "numero_misure_necessarie"=w341:u16)
        n168 = Format Into String(format string="%d/%d", error in=w329, w331, w333) -> (resulting string=w330:string, error out=w328:errorcluster)  [unwired: 1 in]
        n169 = Format Into String(format string="%d/%d", error in=w328, w340, w341) -> (resulting string=w343:string, error out=w345:errorcluster)  [unwired: 1 in]
        n170 = Bundle By Name(cluster=w352, "ByteGSAPIBase in"=w350, "Calibrations"=w346, "Misurazioni"=w348, "Misurazioni index"=w332, "Misurazioni n"=w343, "Misure effettuate"=w340, "Calibrations"=w330) -> (w351:T7)
      }
      frame "CheckTotalMisurations" {
        n171 = Unbundle By Name(w370) -> ()  [unwired: 1 out]
        n172 = Unbundle By Name(w367) -> ("Calibrations"=w376:T3, "Cal Index"=w365:i32, "Misure effettuate"=w364:i32)
        n173 = Unbundle By Name(w376) -> ("controls"=w375:T8)
        n174 = Index Array(array=w375, index=w365) -> (element=w374:T9)
        n175 = Unbundle By Name(w374) -> ("numero_misure_necessarie"=w373:u16)
        n176 = Less Or Equal?(x=w373, y=w364) -> (x <= y?=w372:bool)
        n177 = case shown="True" w372 {
          tunnel: [CalibrationStates."StartCalibration" w388] -> w371
          tunnel: w369 -> [w378 w397]
          tunnel: [w378 w383] -> w368
          tunnel: w367 -> [w377 w399]
          tunnel: [w377 w394] -> w366
          tunnel: w365 -> [_ _]
          frame False {
          }
          frame True {
            n178 = Unbundle By Name(w399) -> ("Misure effettuate"=w401:i32, "Cal Index"=w392:i32, "Waveform Chart"=w396:refnum<vi>, "Calibrations"=w405:T3)
            n179 = Unbundle By Name(w405) -> ("controls"=w393:T8)
            n180 = Index Array(array=w393, index=w392) -> (element=w404:T9)
            n181 = Unbundle By Name(w404) -> ("numero_misure_necessarie"=w403:u16)
            n182 = property class="WFChart (strict)"(reference=w396, error in=w397, "History Data"=dbl[] []) -> (error out=w395:errorcluster)  [unwired: 1 out]
            n183 = Less Or Equal?(x=w403, y=w401) -> (x <= y?=w402:bool)
            n184 = case shown="True" w402 {
              tunnel: w392 -> [w411 w416]
              tunnel: [w411 w415] -> w409
              tunnel: w401 -> [w410 _]
              tunnel: [w410 w412] -> w400
              tunnel: w393 -> [_ w414]
              frame False {
              }
              frame True {
                n185 = Increment(x=w416) -> (x+1=w415:i32)
                n186 = Index Array(array=w414, index=w415) -> (element=w413:T9)
                n187 = Unbundle By Name(w413) -> ("numero_misure_effettuate"=w412:u32)
              }
            }
            n188 = Array Size(array=w393) -> (size(s)=w380:i32)
            n189 = Decrement(x=w380) -> (x-1=w387:i32)
            n190 = call "MisurazioniString.vi"("error in (no error)"=w395, "index"=w409, "Calibration data"=w405) -> ("error out"=w384:errorcluster, "index"=w381:i32, "String"=w408:string)  [unwired: 6 in]
            n191 = Less Or Equal?(x=w387, y=w392) -> (x <= y?=w391:bool)
            n192 = Increment(x=w381) -> (x+1=w385:i32)
            n193 = Format Into String(format string="%d/%d", error in=w384, w385, w380) -> (resulting string=w382:string, error out=w383:errorcluster)  [unwired: 1 in]
            n194 = Bundle By Name(cluster=w399, "Misure effettuate"=w400, "Cal Index"=w409, "Misurazioni"=w408, "Misurazioni index"=w381, "Id Failed"=u32 0, "Failed?"=FALSE, "Calibrations"=w382) -> (w394:T7)
            n195 = Select(t=CalibrationStates."AllowApprove", s=w391, f=CalibrationStates."CheckTotalMisurations") -> (s? t:f=w388:T2)
          }
        }
      }
      frame "StartCalibration" {
        n196 = Unbundle By Name(w432) -> ("Outcome"=w431:refnum<vi>, "Avanti"=w420:refnum<vi>, "Repeat"=w417:refnum<vi>)
        n197 = Build Array(w420, w417) -> (w422:refnum<vi>[])
        n198 = property class="Str"(reference=w431, error in=w428, "Text.BGColor"=u32 9678034 ("Text.Text Colors:BG Color")) -> (error out=w429:errorcluster)  [unwired: 1 out]
        n199 = Unbundle By Name(w443) -> ("Calibrations"=w447:T3, "New Val"=w440:dbl, "Cal Index"=w427:i32, "Misure effettuate"=w424:i32)  [unwired: 1 out]
        n200 = call "DisableControls.vi"("Visible"=FALSE, "Controls"=w422) -> ()  [unwired: 9 in, 1 out]
        n201 = Unbundle By Name(w447) -> ("controls"=w419:T8)
        n202 = call "FGVTimer.vi"("error in"=w429) -> ("error out"=w436:errorcluster, "Elapsed?"=w444:bool)  [unwired: 8 in, 1 out]
        n203 = Index Array(array=w419, index=w427) -> (element=w446:T9)
        n204 = Unbundle By Name(w446) -> ("riferimento_obiettivo"=w438:dbl)
        "Reference value" <- w438
        n205 = Index Array(array=w419, index=w427) -> (element=w426:T9)
        n206 = Unbundle By Name(w426) -> ("numero_misure_necessarie"=w425:u16)
        n207 = case shown="False" w444 {
          tunnel: w438 -> [w454 _]
          tunnel: [CalibrationStates."StartCalibration" CalibrationStates."ManageCalibration"] -> w441
          tunnel: [w448 w457] -> w439
          tunnel: w440 -> [_ w457]
          frame False {
            n208 = Quotient & Remainder(x=w454, y=10.0) -> (floor(x/y)=w453:dbl)  [unwired: 1 out]
            n209 = Add(x=w454, y=w453) -> (x+y=w452:dbl)
            n210 = Subtract(x=w454, y=w453) -> (x-y=w449:dbl)
            n211 = To Quad Integer(1:w452) -> (0:w451:i64)
            n212 = To Quad Integer(1:w449) -> (0:w450:i64)
            n213 = call-poly <vilib>:"Random Number (Range).vi"("lower bound (-100)"=w450, "upper bound (100)"=w451) -> ("number"=w448:i64)  [unwired: 9 in]
            "Waveform Chart" <- w448
          }
          frame True {
          }
        }
        "Measured value" <- w439
        n214 = Increment(x=w424) -> (x+1=w423:i32)
        n215 = Format Into String(format string="%d/%d", error in=w436, w423, w425) -> (resulting string=w435:string, error out=w418:errorcluster)  [unwired: 1 in]
        n216 = Bundle By Name(cluster=w443, "Next State"=w441, "New Val"=w439, "Misurazioni n"=w435, "Stato"="Executing calibration", "Esito"="...") -> (w442:T7)
      }
      frame "ManageCalibration" {
        n217 = Unbundle By Name(w479) -> ("ByteGSAPIBase in"=w482:refnum<class "ByteGSAPIBase.lvclass">, "Calibrations.controls"=w485:T8, "New Val"=w481:dbl, "Id Failed"=w477:u32, "Failed?"=w474:bool, "Cal Index"=w464:i32, "Misure effettuate"=w462:i32)
        n218 = Unbundle By Name(w471) -> ("Repeat"=w460:refnum<vi>, "Avanti"=w461:refnum<vi>, "Outcome"=w468:refnum<vi>)
        n219 = Index Array(array=w485, index=w464) -> (element=w484:T9)
        n220 = Unbundle By Name(w484) -> ("id"=w483:u16, "riferimento_obiettivo"=w480:dbl)
        n221 = disable-structure shown="Enabled" {
          disable-tunnel: w483 -> [w524 _]
          disable-tunnel: w482 -> [w523 w542]
          disable-tunnel: w481 -> [w522 w544]
          disable-tunnel: w480 -> [w521 w545]
          disable-tunnel: w465 -> [w520 w543]
          disable-tunnel: [w516 w543] -> w467
          disable-tunnel: w477 -> [w514 _]
          disable-tunnel: [w513 w542] -> w476
          disable-tunnel: [w512 _] -> w475
          disable-tunnel: w474 -> [w511 _]
          disable-tunnel: [w509 w540] -> w463
          frame Enabled {
            n222 = case shown="True" w511 {
              tunnel: w523 -> [w531 w539]
              tunnel: w521 -> [w530 w532]
              tunnel: w522 -> [w529 w537]
              tunnel: w520 -> [w528 w538]
              tunnel: [w527 w535] -> w519
              tunnel: w524 -> [w525 w534]
              tunnel: [w526 w536] -> w518
              tunnel: [w525 w534] -> w517
              tunnel: w514 -> [_ w533]
              frame False {
                n223 = call-dynamic "AddMeasurement.vi"("measurement-group-id"=w525, "error in (no error)"=w528, "instrument measure"=w529, "reference measure"=w530, "ByteGSAPIBase in"=w531) -> ("error out"=w527:errorcluster, "ByteGSAPIBase out"=w526:refnum<class "ByteGSAPIBase.lvclass">)  [unwired: 4 in, 1 out]
              }
              frame True {
                n224 = call-dynamic "EditMeasurement.vi"("reference measure"=w532, "error in (no error)"=w538, "instrument measure"=w537, "measurement-id"=w533, "ByteGSAPIBase in"=w539) -> ("error out"=w535:errorcluster, "ByteGSAPIBase out"=w536:refnum<class "ByteGSAPIBase.lvclass">)  [unwired: 4 in, 1 out]
              }
            }
            n225 = call-dynamic "MeasGroupResult.vi"("error in (no error)"=w519, "measurement_group_id"=w517, "ByteGSAPIBase in"=w518) -> ("error out"=w516:errorcluster, "measurements"=w515:cluster{"id":u32, "passed":bool}[], "ByteGSAPIBase out"=w513:refnum<class "ByteGSAPIBase.lvclass">)  [unwired: 5 in, 1 out]
            n226 = call "GetResult.vi"("measurements"=w515) -> ("passed"=w510:bool, "id"=w512:u32)  [unwired: 1 in]
            n227 = Not(x=w510) -> (.not. x?=w509:bool)
          }
          frame Disabled {
            n228 = Equal?(x=w545, y=w544) -> (x = y?=w541:bool)
            n229 = Not(x=w541) -> (.not. x?=w540:bool)
          }
        }
        n230 = case shown="True" w463 {
          tunnel: ["PASSED" ("Esito") "FAILED" ("Esito")] -> w469
          tunnel: w468 -> [w502 w506]
          tunnel: w467 -> [w500 w505]
          tunnel: [w499 w504] -> w466
          frame False {
            n231 = property class="Str"(reference=w502, error in=w500, "Text.BGColor"=u32 5558784 ("Text.Text Colors:BG Color")) -> (error out=w499:errorcluster)  [unwired: 1 out]
          }
          frame True {
            n232 = property class="Str"(reference=w506, error in=w505, "Text.BGColor"=u32 16737380 ("Text.Text Colors:BG Color")) -> (error out=w504:errorcluster)  [unwired: 1 out]
          }
        }
        n233 = case shown="True" w463 {
          tunnel: w462 -> [w493 w498]
          tunnel: [w492 w498] -> w459
          tunnel: w460 -> [w487 w495]
          tunnel: w461 -> [w486 w494]
          frame False {
            n234 = Build Array(w486) -> (w489:refnum<vi>[])
            n235 = Build Array(w487) -> (w491:refnum<vi>[])
            n236 = Increment(x=w493) -> (x+1=w492:i32)
            n237 = call "DisableControls.vi"("Visible"=FALSE, "Controls"=w491) -> ()  [unwired: 9 in, 1 out]
            n238 = call "DisableControls.vi"("Visible"=TRUE, "Controls"=w489) -> ()  [unwired: 9 in, 1 out]
          }
          frame True {
            n239 = Build Array(w495, w494) -> (w497:refnum<vi>[])
            n240 = call "DisableControls.vi"("Visible"=TRUE, "Controls"=w497) -> ()  [unwired: 9 in, 1 out]
          }
        }
        n241 = Bundle By Name(cluster=w479, "ByteGSAPIBase in"=w476, "Id Failed"=w475, "Failed?"=w463, "Next State"=CalibrationStates."Idle", "Stato"="Calibration executed", "Esito"=w469, "Misure effettuate"=w459) -> (w478:T7)
      }
      frame "AllowApprove" {
        n242 = Unbundle By Name(w555) -> ("Repeat"=w554:refnum<vi>, "Approvation"=w552:refnum<vi>, "Avanti"=w553:refnum<vi>)
        n243 = Unbundle By Name(w546) -> ("Calibrations.controls"=w547:T8, "Misure effettuate"=w551:i32, "Cal Index"=w550:i32)
        n244 = Array Size(array=w547) -> (size(s)=w562:i32)
        n245 = Decrement(x=w562) -> (x-1=w561:i32)
        n246 = Index Array(array=w547, index=w550) -> (element=w560:T9)
        n247 = Less Or Equal?(x=w561, y=w550) -> (x <= y?=w557:bool)
        n248 = Unbundle By Name(w560) -> ("numero_misure_necessarie"=w559:u16)
        n249 = Equal?(x=w551, y=w559) -> (x = y?=w558:bool)
        n250 = And(x=w558, y=w557) -> (x .and. y?=w556:bool)
        n251 = case shown="True" w556 {
          tunnel: w552 -> [_ w566]
          tunnel: w553 -> [_ w569]
          tunnel: w554 -> [_ w563]
          frame False {
          }
          frame True {
            n252 = Build Array(w566) -> (w565:refnum<vi>[])
            n253 = Build Array(w569, w563) -> (w568:refnum<vi>[])
            n254 = call "DisableControls.vi"("Visible"=TRUE, "Controls"=w565) -> ()  [unwired: 9 in, 1 out]
            n255 = call "DisableControls.vi"("Visible"=FALSE, "Controls"=w568) -> ()  [unwired: 9 in, 1 out]
          }
        }
      }
      frame "Approve" {
        n256 = Unbundle By Name(w580) -> ("Cancel"=w570:refnum<vi>, "Approvation"=w579:refnum<vi>)
        n257 = Build Array(w579) -> (w578:refnum<vi>[])
        n258 = call "DisableControls.vi"("Visible"=FALSE, "Controls"=w578) -> ()  [unwired: 9 in, 1 out]
        n259 = disable-structure shown="Enabled" {
          disable-tunnel: w583 -> [w584 w595]
          disable-tunnel: w582 -> [w587 w594]
          disable-tunnel: [w586 w595] -> w576
          disable-tunnel: [w585 w594] -> w572
          frame Enabled {
            n260 = in-place {
              in-place-border: w584 -> [w591]
              in-place-border: [w590] -> w585
              in-place-border: w587 -> [w588]
              n261 = in-place-cluster #2(w584) -> ("ByteGSAPIBase in"=w593:refnum<class "ByteGSAPIBase.lvclass">)
              n262 = Unbundle By Name(w591) -> ("Selected Slug"=w589:i32)
              n263 = call-dynamic "RequestApproval.vi"("error in (no error)"=w588, "calibration-id"=w589, "ByteGSAPIBase in"=w593) -> ("error out"=w590:errorcluster, "ByteGSAPIBase out"=w592:refnum<class "ByteGSAPIBase.lvclass">)  [unwired: 6 in, 1 out]
              n264 = in-place-cluster #2("ByteGSAPIBase in"=w592) -> (w586:T7)
            }
          }
          frame Disabled {
          }
        }
        n265 = property class="Bool"(reference=w570, error in=w572, "BoolText.Text"="RESTART" ("Boolean Text.Text")) -> (error out=w571:errorcluster)  [unwired: 1 out]
        n266 = Bundle By Name(cluster=w576, "Stato"="Request of approval sent") -> (w575:T7)
      }
    }
    n267 = Unbundle By Name(w42) -> ("Misurazioni"=→"Calibration n.":string, "Misurazioni n"=→"Calibration n.":string, "Stato"=→"Status":string, "Esito"=→"Outcome":string, "Calibrations"=→"Calibrations":string)
    n268 = Or(x=w33, y=w34) -> (x .or. y?=w35:bool)
  }
